vi "Split Matrix.vi"(11 "Current":T1 format="%.3f") -> (0 "Position":dbl[](array[numeric]), 1 "Tangent":dbl[](array[numeric]), 2 "Approach":dbl[](array[numeric]), 3 "Normal":dbl[](array[numeric]))   [LabVIEW 2013]
uses:
  <vilib>/Analysis/Matrix/Datatypes/RealMatrix.ctl
  <vilib>/Analysis/Matrix/NI_Matrix.lvlib
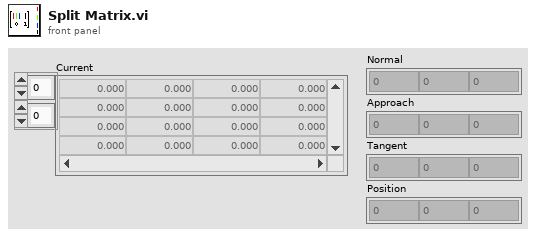
[diagram p1: front panel]
types:
  T1 = typedef "NI_Matrix.lvlib/RealMatrix.ctl" = dbl[][]
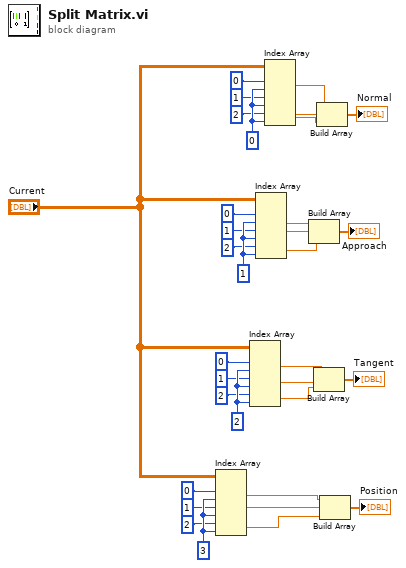
[diagram p0: block diagram]
diagram:
  w16 = 0 ("index (col)")
  w20 = 1 ("index (col)")
  w24 = 2 ("index (col)")
  w32 = 3 ("index (col)")
  n1 = Index Array(array="Current", index (row) #1=0 ("index (row)"), index (col) #1=w32, index (row) #2=1 ("index (row)"), index (col) #2=w32, index (row) #3=2 ("index (row)"), index (col) #3=w32) -> (element #1=w29:dbl, element #2=w28:dbl, element #3=w27:dbl)
  n2 = Index Array(array="Current", index (row) #1=0 ("index (row)"), index (col) #1=w24, index (row) #2=1 ("index (row)"), index (col) #2=w24, index (row) #3=2 ("index (row)"), index (col) #3=w24) -> (element #1=w9:dbl, element #2=w8:dbl, element #3=w7:dbl)
  n3 = Index Array(array="Current", index (row) #1=0 ("index (row)"), index (col) #1=w20, index (row) #2=1 ("index (row)"), index (col) #2=w20, index (row) #3=2 ("index (row)"), index (col) #3=w20) -> (element #1=w5:dbl, element #2=w4:dbl, element #3=w6:dbl)
  n4 = Index Array(array="Current", index (row) #1=0 ("index (row)"), index (col) #1=w16, index (row) #2=1 ("index (row)"), index (col) #2=w16, index (row) #3=2 ("index (row)"), index (col) #3=w16) -> (element #1=w1:dbl, element #2=w2:dbl, element #3=w3:dbl)
  n5 = Build Array(w5, w4, w6) -> (→"Approach":dbl[])
  n6 = Build Array(w9, w8, w7) -> (→"Tangent":dbl[])
  n7 = Build Array(w1, w2, w3) -> (→"Normal":dbl[])
  n8 = Build Array(w29, w28, w27) -> (→"Position":dbl[])
